vi "PH_Interaction.select instances of multiple classes from database.vi"(3 "error in (no error)":errorcluster, 4 "Classes Input":string[](array[string])) -> (0 "error out":errorcluster, 1 "Query Result":cluster{"Object Name":string, "Class":string}[](array[cluster]))   [LabVIEW 2014, in "PH_Common.lvlib"]
doc: "This VI retrieves data from a DataBase via SQL (tested with MS Access). \n\nThe result is given out as an array of clusters. The clusters contain the object name and the class where they belonging to as string."
uses:
  CS_Core/CSSystem/CoreDefs/CoreDefs.error_type.ctl
  PH_Common.lvlib
  CS_Core/CSSystem/CoreLib/CoreLib.lvlib
  CS_Core/CSSystem/CSSystemLib/CSSystemLib.lvlib
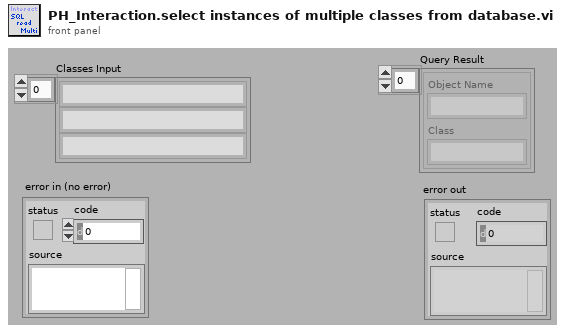
[diagram p1: front panel]
types:
  T1 = typedef "CoreDefs.error_type.ctl" = enum16{"no error", "can't load process", "can't unload process", "process does not exist", "can't install process", "can't remove process", "unknown function", "time out", "can't execute function", "duplicate queue name", "super not found", "caller queue invalid", "can't ping process", "unknown error", "VISA Error", "VISA timeout", "GPIB timeout", "GPIB error", "communication error", "data type mismatch", "can't read data from OPC server", "can't write data to OPC server", "OET error", "function not implemented", "process already exists", "invalid Shared Variable name", "error writing Shared Variable", "error reading Shared Variable", "invalid client name", "corrupt database", "unknown class", "call not authorized", "parameter out of range", "OET timeout: can't get data to modify", "invalid queue name", "requested operation incompatible with current state", "event undefined", "event disabled", "state undefined", "caller is not a friend", "EventBuilder: bad eventID", "EventBuilder: no DAQ devices", "a thread must not stop itself", "UNUSED ELEMENT4", "DiscArchiver: eventData incomplete", "DiscArchiver: eventData does not belong to run", "DiscArchiver: can't open file", "DiscArchiver: can't write to file", "DiscArchiver: available disc space low", "can't acquire semaphore", "error reading data from database", "notifier object is not existing", "can't register process", "can't unregister process", "illegal event type", "object disabled", "object already exists", "can't change state", "Instrument not found", "no connection to remote node", "invalid reference", "N/A", "UNUSED ELEMENT 1", "element not found", "illegal TCP/IP connection detected", "object does not exist", "invalid access ID", "unknown CS system", "invalid privilige", "unsupported data type", "unsupported server type", "IO server already exists", "Shared Variable already exists"}
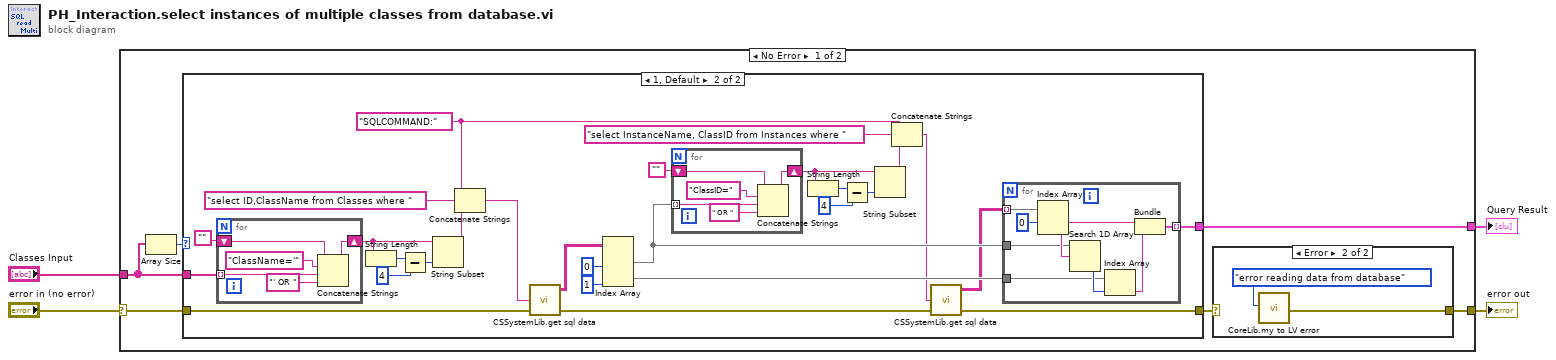
[diagram p0: block diagram]
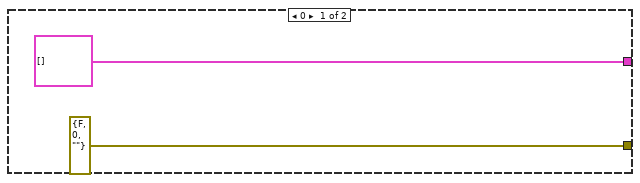
[diagram p2: hidden frame]
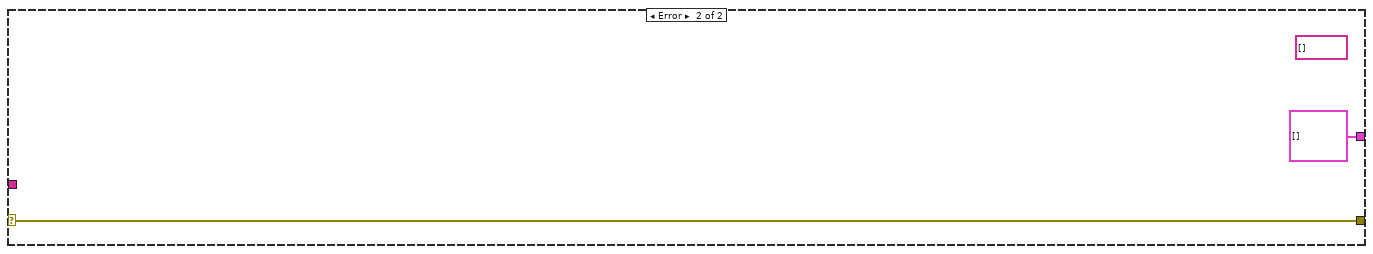
[diagram p4: hidden frame]
diagram:
  n1 = case shown="No Error" "error in (no error)" {
    selector: "error in (no error)" -> [w6 w64]
    tunnel: [w9 w64] -> w4
    tunnel: "Classes Input" -> [w8 _]
    tunnel: [w5 cluster{"Object Name":string, "Class":string}[] []] -> w1
    frame No Error {
      n2 = Array Size(array=w8) -> (size(s)=w7:i32)
      n3 = case shown="1, Default" w7 {
        tunnel: [errorcluster {"status"=FALSE, "code"=0, "source"=""} ("error out") w15] -> w10
        tunnel: w8 -> [_ w32]
        tunnel: w6 -> [_ w40]
        tunnel: [cluster{"Object Name":string, "Class":string}[] [] w14] -> w5
        frame 0 {
        }
        frame 1, Default {
          w13 = "SQLCOMMAND:" ("string")
          n4 = for {
            tunnel: w32 -> [w58] mode=indexing
            shift-right: [w55] -> w35
            shift-left: "" -> [w56]
            n5 = Concatenate Strings(w56, "ClassName='" ("string"), w58, "' OR " ("string")) -> (w55:string)
          }
          n6 = String Length(string=w35) -> (length=w37:i32)
          n7 = Subtract(x=w37, y=4) -> (x-y=w34:i32)
          n8 = String Subset(string=w35, length (rest)=w34) -> (substring=w33:string)  [unwired: 1 out]
          n9 = Concatenate Strings(w13, "select ID,ClassName from Classes where " ("string"), w33) -> (w31:string)
          n10 = call "CSSystemLib.get sql data.vi"("error in (no error)"=w40, "object"=w31) -> ("error out"=w17:errorcluster, "queryResults"=w19:string[][])  [unwired: 1 in, 1 out]
          n11 = Index Array(array=w19, index (col) #1=0 ("disabled index (col)"), index (col) #2=1 ("index (col)")) -> (element #1=w28:string[], element #2=w29:string[])  [unwired: 2 in]
          n12 = for {
            tunnel: w28 -> [w53] mode=indexing
            shift-right: [w50] -> w23
            shift-left: "" -> [w51]
            n13 = Concatenate Strings(w51, "ClassID=" ("string"), w53, " OR " ("string")) -> (w50:string)
          }
          n14 = String Length(string=w23) -> (length=w25:i32)
          n15 = Subtract(x=w25, y=4) -> (x-y=w22:i32)
          n16 = String Subset(string=w23, length (rest)=w22) -> (substring=w27:string)  [unwired: 1 out]
          n17 = Concatenate Strings(w13, "select InstanceName, ClassID from Instances where " ("string"), w27) -> (w18:string)
          n18 = call "CSSystemLib.get sql data.vi"("error in (no error)"=w17, "object"=w18) -> ("error out"=w15:errorcluster, "queryResults"=w16:string[][])  [unwired: 1 in, 1 out]
          n19 = for {
            tunnel: w16 -> [w49] mode=indexing
            tunnel: w28 -> [w46]
            tunnel: w29 -> [w44]
            tunnel: [w41] -> w14 mode=indexing
            n20 = Index Array(array=w49, index #1=0 ("index")) -> (element #1=w43:string, element #2=w47:string)  [unwired: 1 in]
            n21 = Search 1D Array(1D array=w46, element=w47) -> (index of element=w45:i32)  [unwired: 1 out]
            n22 = Index Array(array=w44, index=w45) -> (element=w42:string)
            n23 = Bundle(w43, w42) -> (w41:cluster{string, string})  [unwired: 1 out]
          }
        }
      }
      n24 = case shown="Error" w10 {
        selector: w10 -> [w60 _]
        tunnel: [w60 w61] -> w9
        frame No Error {
        }
        frame Error {
          n25 = call "CoreLib.my to LV error.vi"("ErrorTypes"=CoreDefs.error_type."error reading data from database") -> ("myErrorCluster"=w61:errorcluster)  [unwired: 17 in, 1 out]
        }
      }
    }
    frame Error {
      (unwired) string[] []
    }
  }
  "error out" <- w4
  "Query Result" <- w1
